vi "Warning Dialog.vi"(11 "Path":path) -> (3 "Continue?":bool)   [LabVIEW 2019, in "Shared.lvlib"]
uses:
  Shared.lvlib
  Panther Dashboard/Panther Dashboard.lvlib
panel:
  in  "Cancel":bool
  in  "Continue":bool
  out "Message":string
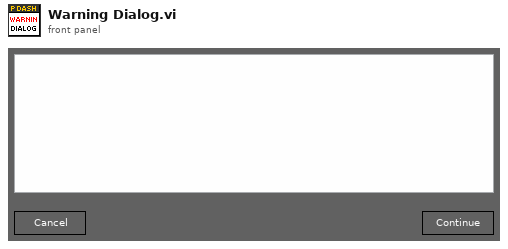
[diagram p1: front panel]
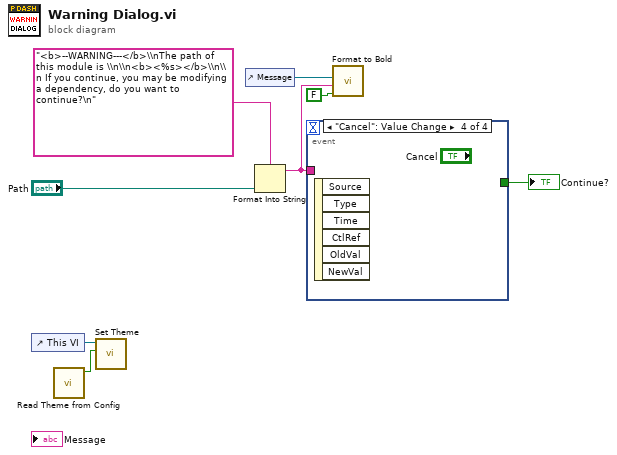
[diagram p0: block diagram]
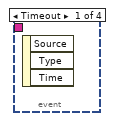
[diagram p2: hidden frame]
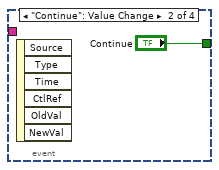
[diagram p3: hidden frame]
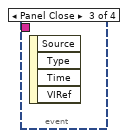
[diagram p4: hidden frame]
diagram:
  n1 = control-ref of="This VI"() -> (w7:refnum<vi>)
  n2 = call "Read Theme from Config.vi"() -> ("Theme"=w6:bool)  [unwired: 10 in, 1 out]
  n3 = call "Set Theme.vi"("Dark?"=w6, "VI in"=w7) -> ()  [unwired: 10 in]
  n4 = control-ref of="Message"() -> (w5:refnum<vi>)
  n5 = Format Into String(format string="<b>--WARNING---</b>\\nThe path of this module is \\n\\n<b><%s></b>\\n\\n If you continue, you may be modifying a dependency, do you want to continue?\n" ("message"), "Path") -> (resulting string=w1:string)  [unwired: 2 in, 1 out]
  n6 = event shown="[3] \"Cancel\": Value Change" {
    selector: _ -> [_ _ _ _]
    dyn-events: _ -> [_ _ _ _]
    timeout: _ -> [_ _ _ _]
    tunnel: [_ "Continue" _ _] -> w2
    tunnel: w1 -> [_ _ _ _]
    event Timeout {
      n7 = event-data() -> ()  [unwired: 1 in, 3 out]
    }
    event "Continue": Value Change {
      n8 = event-data() -> ()  [unwired: 1 in, 6 out]
    }
    event Panel Close {
      n9 = event-data() -> ()  [unwired: 1 in, 4 out]
    }
    event "Cancel": Value Change {
      n10 = event-data() -> ()  [unwired: 1 in, 6 out]
    }
  }
  "Continue?" <- w2
  n11 = call "Format to Bold.vi"("Adjust Height?"=FALSE, "String Value"=w1, "String Ref"=w5) -> ()  [unwired: 9 in]
